vi "Convert float to payload.vi"(0 "FloatNumber":sgl) -> (14 "Converted Payload":u8[](array[numeric]) format="%.0x")   [LabVIEW 2023]
panel:
  out "Float out":sgl
  in  "Byte4":u8=18 format="%.0x"
  in  "Byte3":u8=160 format="%.0x"
  in  "Byte2":u8=51 format="%.0x"
  in  "Byte1":u8=66 format="%.0x"
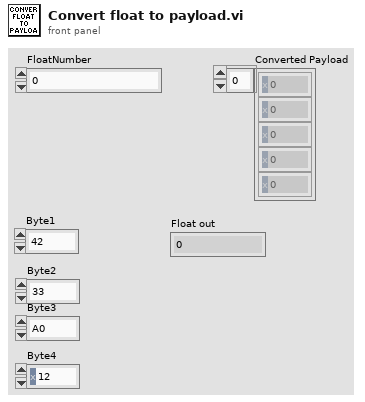
[diagram p1: front panel]
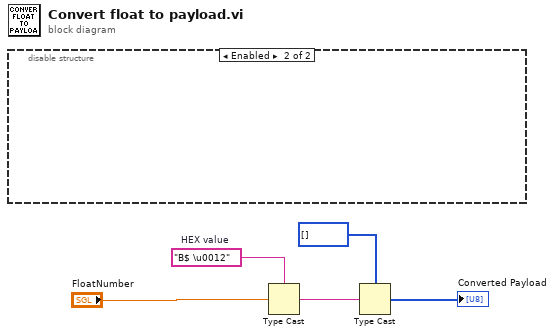
[diagram p0: block diagram]
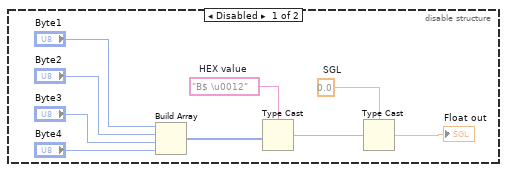
[diagram p2: hidden frame]
diagram:
  w5 = "B$ \u0012"  # HEX value
  n1 = disable-structure shown="Enabled" {
    frame Disabled {
      w14 = sgl 0.0  # SGL
      w13 = "B$ \u0012"  # HEX value
      n2 = Build Array("Byte1", "Byte2", "Byte3", "Byte4") -> (w11:u8[])
      n3 = Type Cast(type=w13, x=w11) -> (*(type *) &x=w12:string)
      n4 = Type Cast(type=w14, x=w12) -> (*(type *) &x=→"Float out":sgl)
    }
    frame Enabled {
    }
  }
  n5 = Type Cast(type=w5, x="FloatNumber") -> (*(type *) &x=w1:string)
  n6 = Type Cast(type=u8[] [] ("appended array"), x=w1) -> (*(type *) &x=→"Converted Payload":u8[])
